vi "FTW-Actor-Initialized.vi"(0 "FTW Actor Instance":refnum<class "FTW-ActorInstance.lvclass">, 5 "Initialized Response":string, 11 "error in":errorcluster) -> (4 "FTW Actor Instance out":refnum<class "FTW-ActorInstance.lvclass">, 15 "error out":errorcluster)   [LabVIEW 2013, in "FTW-ActorInstance.lvclass"]
uses:
  FTW-ActorInstance.lvclass
  FTW-Actor-FrameworkEvent.ctl
  FTW-ActorInstance.lvclass/FTW-ActorInstance.ctl
  Time/FTW-Time-DisplayFormat-Timestamp.ctl
  Endpoint/FTW-Endpoint.lvclass
  Ether/FTW-Ether.lvclass
panel:
  # "Inputs"
  # "Outputs"
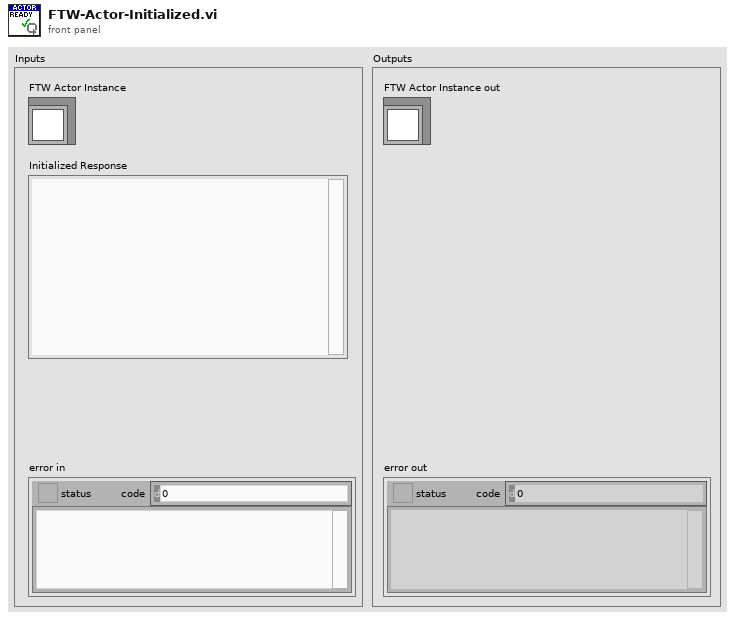
[diagram p1: front panel]
types:
  T1 = typedef "FTW-ActorInstance.lvclass/FTW-Actor-FrameworkEvent.ctl" = enum16{"Instance Initializing", "Instance Initialized", "Instance Job", "Instance Handle Request", "Instance Shutting Down", "Instance Destroyed"}
  T2 = typedef "FTW-Time-DisplayFormat-Timestamp.ctl" = enum16{"YYYY-MM-DDT00:00:00.000Z (ISO-8601)", "YYYY-MM-DDT00-00-00Z (Simple ISO-8601)", "YYYY-MM-DD"}
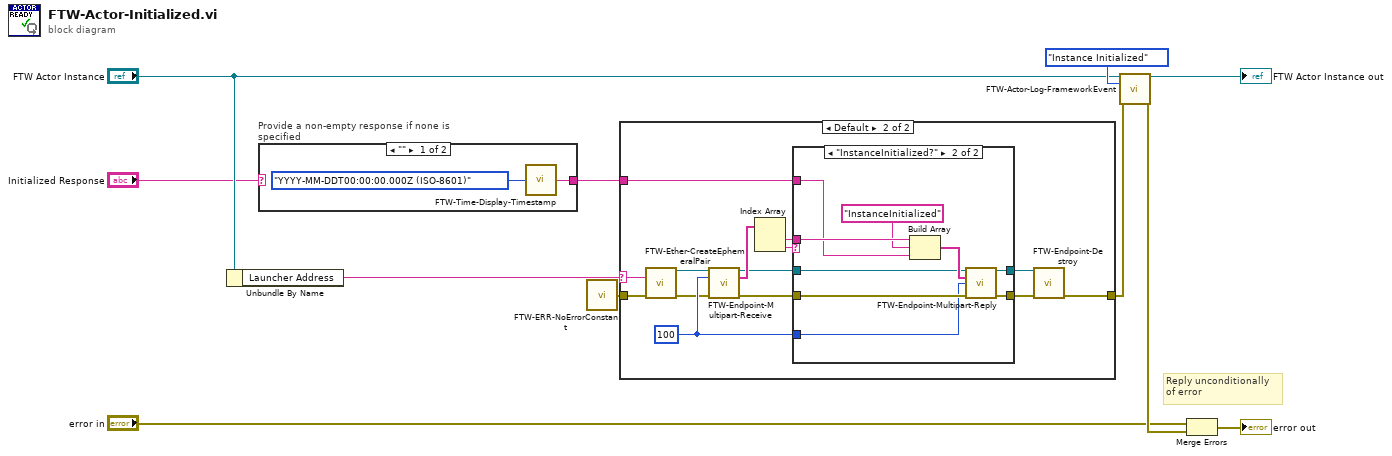
[diagram p0: block diagram]
diagram:
  # "Reply unconditionally\nof error"
  n1 = Unbundle By Name("FTW Actor Instance") -> ("Launcher Address"=w7:string)
  n2 = case "Provide a non-empty response if none is specified" shown="\"\"" "Initialized Response" {
    selector: "Initialized Response" -> [_ w14]
    tunnel: [w13 w14] -> w5
    frame "" {
      n3 = call "FTW-Time-Display-Timestamp.vi"("Format"=FTW-Time-DisplayFormat-Timestamp."YYYY-MM-DDT00:00:00.000Z (ISO-8601)") -> ("Formatted Timestamp"=w13:string)  [unwired: 3 in]
    }
    frame Default {
    }
  }
  n4 = call "FTW-ERR-NoErrorConstant.vi"() -> ("no error"=w4:errorcluster)
  n5 = case shown="Default" w7 {
    selector: w7 -> [_ w16]
    tunnel: w5 -> [_ w24]
    tunnel: [w15 w21] -> w8
    tunnel: w4 -> [w15 w18]
    frame "" {
    }
    frame Default {
      w20 = 100
      n6 = call "FTW-Ether-CreateEphemeralPair.vi"("Requested Ephemeral Address"=w16, "error in"=w18) -> ("Ephemeral Endpoint"=w19:refnum<class "FTW-Endpoint.lvclass">, "error out"=w17:errorcluster)  [unwired: 11 in, 1 out]
      n7 = call-dynamic "FTW-Endpoint-Multipart-Receive.vi"("FTW Endpoint"=w19, "Timeout"=w20, "error in"=w17) -> ("FTW Endpoint out"=w23:refnum<class "FTW-Endpoint.lvclass">, "Message Received"=w28:string[], "error out"=w29:errorcluster)  [unwired: 9 in, 1 out]
      n8 = Index Array(array=w28) -> (element #1=w25:string, element #2=w27:string)  [unwired: 2 in]
      n9 = case shown="\"InstanceInitialized?\"" w27 {
        tunnel: w29 -> [w31 w40]
        tunnel: [w30 w39] -> w26
        tunnel: w25 -> [_ w38]
        tunnel: w24 -> [_ w32]
        tunnel: w23 -> [w30 w36]
        tunnel: [w31 w35] -> w22
        tunnel: w20 -> [_ w34]
        frame Default {
        }
        frame "InstanceInitialized?" {
          n10 = Build Array(w38, "InstanceInitialized" ("element"), w32) -> (w37:string[])
          n11 = call-dynamic "FTW-Endpoint-Multipart-Reply.vi"("FTW Endpoint"=w36, "Multipart Message"=w37, "Timeout"=w34, "error in"=w40) -> ("FTW Endpoint out"=w39:refnum<class "FTW-Endpoint.lvclass">, "error out"=w35:errorcluster)  [unwired: 9 in, 1 out]
        }
      }
      n12 = call-dynamic "FTW-Endpoint-Destroy.vi"("FTW Endpoint"=w26, "error in"=w22) -> ("error out"=w21:errorcluster)  [unwired: 13 in]
    }
  }
  n13 = call "FTW-Actor-Log-FrameworkEvent.vi"("FTW Actor Instance"="FTW Actor Instance", "Framework Event"=FTW-Actor-FrameworkEvent."Instance Initialized", "error in"=w8) -> ("FTW Actor Instance out"=→"FTW Actor Instance out":refnum<class "FTW-ActorInstance.lvclass">, "error out"=w3:errorcluster)  [unwired: 11 in]
  n14 = Merge Errors("error in", w3) -> (→"error out":errorcluster)
